vi "JL_Create_Blink_Expected_LEDs.vi"(5 "SSD":string, 7 "Boolean":bool) -> (8 "Expected LEDs Out":T1={"SSD"="", "Cycle Selection"=enum."Cycle 0", "Bar Selection"=enum."Bar 1", "Temp Setting"=enum."No Heat", "Dryness Level"=enum."Damp", "Time Setting"=enum."Off", "Dryer Status"=enum."Status 1", "Start/Pause"=FALSE, "Pause"=FALSE, "Control Lock"=FALSE, "Sensing"=FALSE, "Clean Filter"=FALSE, "My Cycle"=FALSE, "Delay Dry"=FALSE, "Volume"=FALSE, "Damp Alert"=FALSE, "Ext Tumble"=FALSE, "Decrement"=FALSE, "Increment"=FALSE, "eDry"=FALSE, "Extra Status"=FALSE})   [LabVIEW 2016]
uses:
  type defs/JL Display.ctl
  type defs/Cycle Selection Enum.ctl
  type defs/Bar Enum.ctl
  type defs/Temp Setting Enum.ctl
  type defs/Dryness Enum.ctl
  type defs/Time Enum.ctl
  type defs/Status Enum.ctl
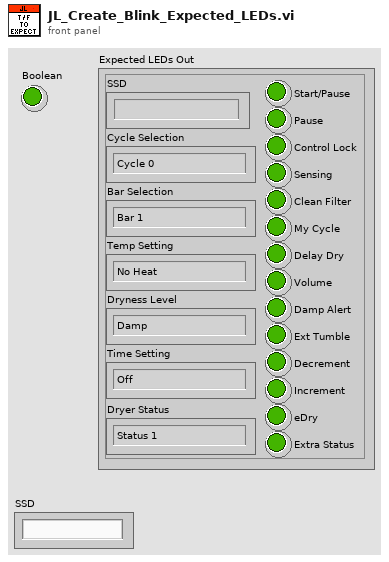
[diagram p1: front panel]
types:
  T1 = typedef "JL Display.ctl" = cluster{"SSD":string, "Cycle Selection":T2, "Bar Selection":T3, "Temp Setting":T4, "Dryness Level":T5, "Time Setting":T6, "Dryer Status":T7, "Start/Pause":bool, "Pause":bool, "Control Lock":bool, "Sensing":bool, "Clean Filter":bool, "My Cycle":bool, "Delay Dry":bool, "Volume":bool, "Damp Alert":bool, "Ext Tumble":bool, "Decrement":bool, "Increment":bool, "eDry":bool, "Extra Status":bool}
  T2 = typedef "Cycle Selection Enum.ctl" = enum16{"Cycle 0", "Cycle 1", "Cycle 2", "Cycle 3", "Cycle 4", "Cycle 5", "Cycle 6", "Cycle 7", "Cycle 8", "Cycle 9", "Cycle 10", "Cycle 11", "Cycle 12", "Cycle 13", "Off", "*Invalid"}
  T3 = typedef "Bar Enum.ctl" = enum16{"Bar 1", "Bar 2", "Bar 3", "Bar 4", "Bar 5", "Off", "*Incorrect*"}
  T4 = typedef "Temp Setting Enum.ctl" = enum16{"Off", "No Heat", "Extra Low", "Low", "Medium", "High", "*Incorrect*"}
  T5 = typedef "Dryness Enum.ctl" = enum16{"Off", "Damp", "Less Dry", "Dry", "More Dry", "Extra Dry", "*Incorrect*"}
  T6 = typedef "Time Enum.ctl" = enum16{"Off", "Default Time 1", "Default Time 2", "Default Time 3", "Default Time 4", "Default Time 5", "*Incorrect*"}
  T7 = typedef "Status Enum.ctl" = enum16{"Status 1", "Status 2", "Status 3", "Status 4", "Status 5", "Status 6", "Off", "*Incorrect*"}
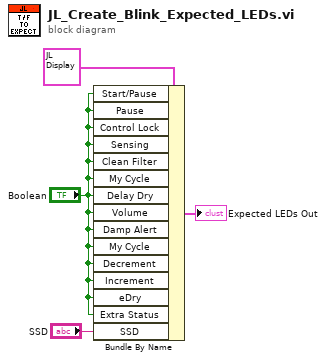
[diagram p0: block diagram]
diagram:
  n1 = Bundle By Name(cluster=T1 {"SSD"="", "Cycle Selection"=enum."Cycle 0", "Bar Selection"=enum."Bar 1", "Temp Setting"=enum."No Heat", "Dryness Level"=enum."Damp", "Time Setting"=enum."Off", "Dryer Status"=enum."Status 1", "Start/Pause"=FALSE, "Pause"=FALSE, "Control Lock"=FALSE, "Sensing"=FALSE, "Clean Filter"=FALSE, "My Cycle"=FALSE, "Delay Dry"=FALSE, "Volume"=FALSE, "Damp Alert"=FALSE, "Ext Tumble"=FALSE, "Decrement"=FALSE, "Increment"=FALSE, "eDry"=FALSE, "Extra Status"=FALSE} ("Expected LEDs Out"), "Start/Pause"="Boolean", "Pause"="Boolean", "Control Lock"="Boolean", "Sensing"="Boolean", "Clean Filter"="Boolean", "My Cycle"="Boolean", "Delay Dry"="Boolean", "Volume"="Boolean", "Damp Alert"="Boolean", "My Cycle"="Boolean", "Decrement"="Boolean", "Increment"="Boolean", "eDry"="Boolean", "Extra Status"="Boolean", "SSD"="SSD") -> (→"Expected LEDs Out":T1)
